vi "DstmEnable.vi"(8 "Error In":errorcluster, 11 "Device Handle":u32) -> (0 "Error Out":errorcluster, 3 "Device Handle":u32)   [LabVIEW 2011, in "LVH-Adept.lvlib" / "DSTM.lvlib"]
uses:
  DSTM.lvlib
  Private/Type Defs/Error.ctl
  Resources/dstm.dll
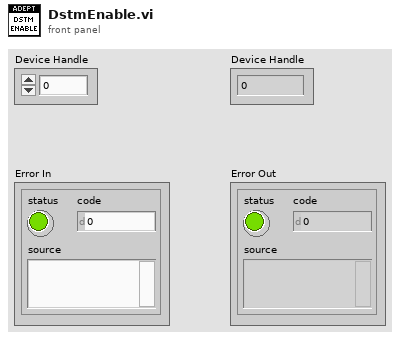
[diagram p1: front panel]
types:
  T1 = typedef "LVH-Adept.lvlib/DSTM.lvlib/Error.ctl" = enum16{"Unknown", "Enable", "Data Transfer", "Disable"}
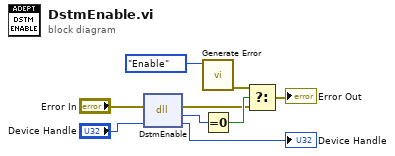
[diagram p0: block diagram]
diagram:
  n1 = dll-call lib="C:/github/labviewhacker/LVH-Adept/LabVIEW/vi.lib/LabVIEW Hacker/Adept/Private/Resources/dstm.dll" fn="DstmEnable"(error in="Error In", "hif"="Device Handle") -> (error out=w2:errorcluster, "Success"=w8:u32, "hif"=→"Device Handle":u32)  [unwired: 2 in, 1 out]
  n2 = call "Generate Error.vi"("DSTM Error"=Error."Enable") -> ("Error Out"=w3:errorcluster)  [unwired: 10 in]
  n3 = Equal To 0?(x=w8) -> (x = 0?=w7:bool)
  n4 = Select(t=w3, s=w7, f=w2) -> (s? t:f=→"Error Out":errorcluster)
